vi "Stereo - Overlay Grid Points.vi"(8 "error in (no error)":errorcluster, 11 "Image in":T1) -> (0 "error out":errorcluster, 1 "Pixel Coordinates":cluster{"X":dbl, "Y":dbl}[](array[cluster]), 2 "Origin Pixel":cluster{"X":dbl, "Y":dbl}, 3 "Image out":T1)   [LabVIEW 2014]
doc: "Analyses the camera model to ensure that all the grids angles are at least 3 degrees apart."
uses:
  <vilib>/vision/Image Controls.llb/IMAQ Image.ctl
  <vilib>/vision/NI_Vision_Development_Module.lvlib
panel:
  # "Overview: Overlay the dots of the grid in red and the origin in green"
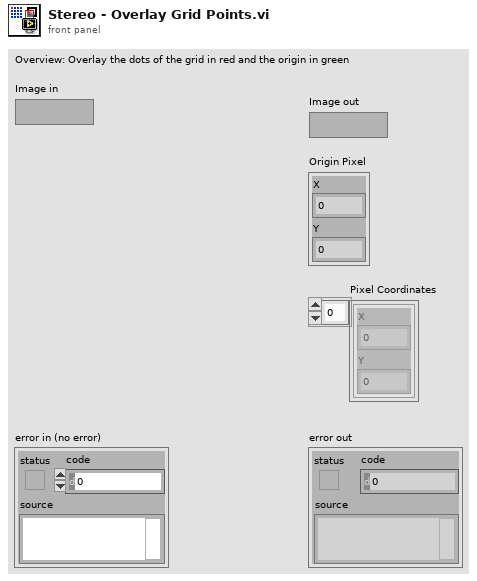
[diagram p1: front panel]
types:
  T1 = typedef "IMAQ Image.ctl" = refnum<image>
  T2 = cluster{"Back Projected Points?":bool, "Undistorted Points?":bool, "Euler Angles?":bool}
  T3 = typedef "Calibration Reference Points.ctl" = cluster{"Pixel Coordinates":cluster{"X":dbl, "Y":dbl}[], "Real World Coordinates":cluster{"X":dbl, "Y":dbl}[], "Unit":T4, "Image Size":cluster{"X":u32, "Y":u32}}
  T4 = typedef "Image Unit" = enum32{"Undefined", "Angström", "Micrometer", "Millimeter", "Centimeter", "Meter", "Kilometer", "Microinch", "Inch", "Feet", "Nautical miles", "Standard miles", "Steps"}
  T5 = cluster{"Origin Pixel":cluster{"X":sgl, "Y":sgl}, "Angle Relative to Horizontal (deg)":sgl, "Axis Reference":u32}
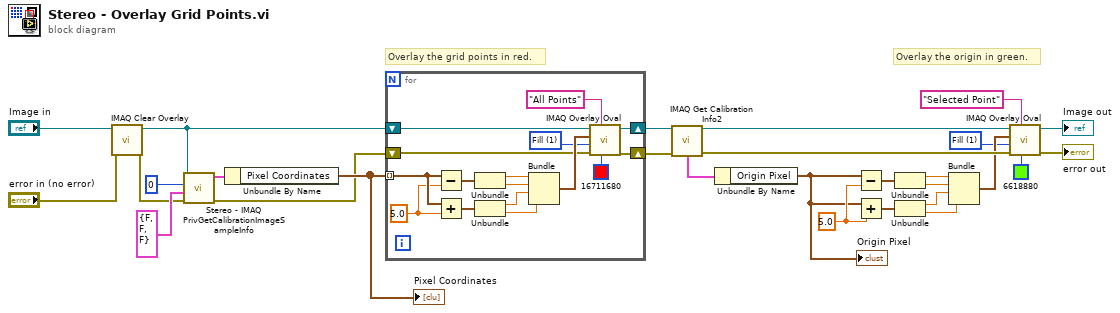
[diagram p0: block diagram]
diagram:
  w3 = u32 1 items=["Frame", "Fill"] ("Drawing Mode (Frame)")
  w25 = sgl 5.0 ("X")
  # "Overlay the grid points in red."
  # "Overlay the origin in green."
  n1 = call "IMAQ Clear Overlay"("error in (no error)"="error in (no error)", "Image"="Image in") -> ("error out"=w9:errorcluster, "Image Out"=w11:T1)  [unwired: 8 in]
  n2 = call "Stereo - IMAQ PrivGetCalibrationImageSampleInfo.vi"("error in (no error)"=w9, "Options"=T2 {"Back Projected Points?"=FALSE, "Undistorted Points?"=FALSE, "Euler Angles?"=FALSE}, "Index"=0, "Template Image"=w11) -> ("error out"=w13:errorcluster, "Reference Points"=w20:T3)  [unwired: 6 out]
  n3 = Unbundle By Name(w20) -> ("Pixel Coordinates"=w19:cluster{"X":dbl, "Y":dbl}[])
  "Pixel Coordinates" <- w19
  n4 = for {
    tunnel: w19 -> [w44] mode=indexing
    shift-right: [w33] -> w23
    shift-left: w11 -> [w41]
    shift-right: [w30] -> w14
    shift-left: w13 -> [w29]
    w31 = 5.0 ("X")
    w35 = u32 1 items=["Frame", "Fill"] ("Drawing Mode (Frame)")
    n5 = Subtract(x=w44, y=w31) -> (x-y=w43:cluster{"X":dbl, "Y":dbl})
    n6 = Add(x=w44, y=w31) -> (x+y=w42:cluster{"X":dbl, "Y":dbl})
    n7 = Unbundle(w43) -> ("X"=w40:dbl, "Y"=w39:dbl)
    n8 = Unbundle(w42) -> ("X"=w37:dbl, "Y"=w38:dbl)
    n9 = Bundle("X"=w40, "Y"=w39, "X"=w37, "Y"=w38) -> (w36:cluster{"X":dbl, "Y":dbl, "X":dbl, "Y":dbl})  [unwired: 1 out]
    n10 = call "IMAQ Overlay Oval"("Color"=u32 16711680, "Group"="All Points", "error in (no error)"=w29, "Drawing Mode (Frame)"=w35, "Bounding Rectangle"=w36, "Image"=w41) -> ("error out"=w30:errorcluster, "Image Out"=w33:T1)  [unwired: 4 out]
  }
  n11 = call "IMAQ Get Calibration Info2"("Calibration Template Image"=w23, "error in (no error)"=w14) -> ("Calibration Template Image (duplicate)"=w24:T1, "Calibration Axis Info"=w28:T5, "error out"=w15:errorcluster)  [unwired: 1 in, 10 out]
  n12 = Unbundle By Name(w28) -> ("Origin Pixel"=w18:cluster{"X":sgl, "Y":sgl})
  "Origin Pixel" <- w18
  n13 = Subtract(x=w18, y=w25) -> (x-y=w27:cluster{"X":sgl, "Y":sgl})
  n14 = Add(x=w18, y=w25) -> (x+y=w26:cluster{"X":sgl, "Y":sgl})
  n15 = Unbundle(w27) -> ("X"=w8:sgl, "Y"=w7:sgl)
  n16 = Unbundle(w26) -> ("X"=w5:sgl, "Y"=w6:sgl)
  n17 = Bundle("X"=w8, "Y"=w7, "X"=w5, "Y"=w6) -> (w4:cluster{"X":sgl, "Y":sgl, "X":sgl, "Y":sgl})  [unwired: 1 out]
  n18 = call "IMAQ Overlay Oval"("Color"=u32 6618880, "Group"="Selected Point", "error in (no error)"=w15, "Drawing Mode (Frame)"=w3, "Bounding Rectangle"=w4, "Image"=w24) -> ("error out"=→"error out":errorcluster, "Image Out"=→"Image out":T1)  [unwired: 4 out]
